vi "Change Endianness (U64).vi"(11 "number in":u64 format="%064b") -> (3 "byte-reversed number out":u64 format="%064b")   [LabVIEW 2016, in "GE 5565PIORC Old.lvclass"]
uses:
  GE 5565PIORC Old.lvclass
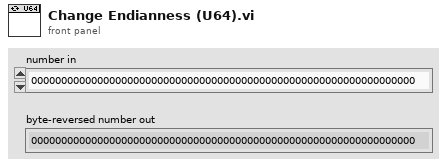
[diagram p1: front panel]
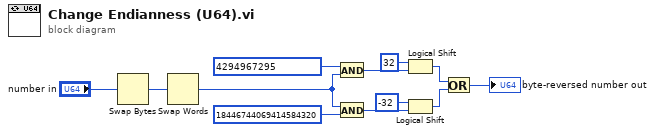
[diagram p0: block diagram]
diagram:
  n1 = Swap Bytes(anything="number in") -> (byte swapped=w6:u64)
  n2 = Swap Words(1:w6) -> (0:w1:u64)
  n3 = And(x=u64 4294967295 ("number in"), y=w1) -> (x .and. y?=w8:u64)
  n4 = And(x=w1, y=u64 18446744069414584320 ("number in")) -> (x .and. y?=w11:u64)
  n5 = Logical Shift(y=i16 32, x=w8) -> (x << y=w5:u64)
  n6 = Logical Shift(y=i16 -32, x=w11) -> (x << y=w4:u64)
  n7 = Or(x=w5, y=w4) -> (x .or. y?=→"byte-reversed number out":u64)
